vi "v_movematrix.vi"(1 "xyz":dbl[](array[numeric])=[0.0, 0.0, 0.0]) -> (0 "matrix":dbl[][](array[numeric])=[[1.0, 0.0, 0.0, 0.0], [0.0, 1.0, 0.0, 0.0], [0.0, 0.0, 1.0, 0.0], [0.0, 0.0, 0.0, 1.0]])   [LabVIEW 2011]
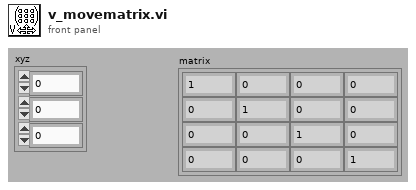
[diagram p1: front panel]
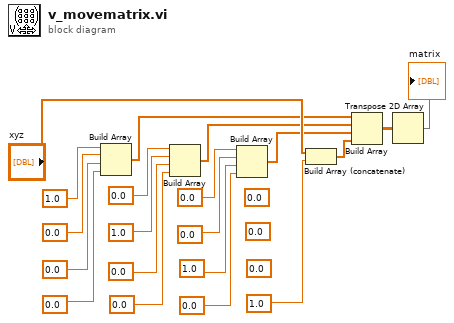
[diagram p0: block diagram]
diagram:
  (unwired) 0.0
  (unwired) 0.0
  (unwired) 0.0
  n1 = Build Array(1.0, 0.0, 0.0, 0.0) -> (w3:dbl[])
  n2 = Build Array(0.0, 1.0, 0.0, 0.0) -> (w2:dbl[])
  n3 = Build Array(0.0, 0.0, 1.0, 0.0) -> (w1:dbl[])
  n4 = Build Array (concatenate)("xyz", 1.0) -> (w6:dbl[])
  n5 = Build Array(w3, w2, w1, w6) -> (w16:dbl[][])
  n6 = Transpose 2D Array(2D array=w16) -> (transposed array=→"matrix":dbl[][])
